vi "Ctor.vi"(8 "error in (no error)":errorcluster) -> (0 "error out":errorcluster, 3 "ByRef Example out":refnum<class "ByRef Example.lvclass">)   [LabVIEW 2012, in "ByRef Example.lvclass"]
uses:
  ByRef Example.lvclass
  Ref Data.ctl
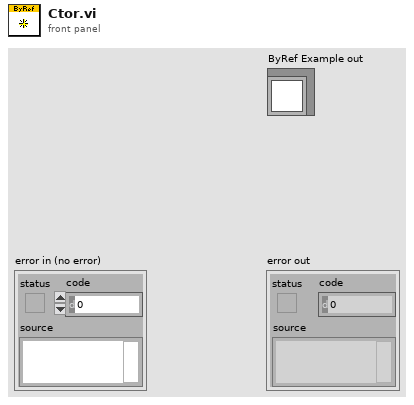
[diagram p1: front panel]
types:
  T1 = typedef "ByRef Example.lvclass/Ref Data.ctl" = cluster{"Boolean":bool, "Numeric":dbl, "String":string}
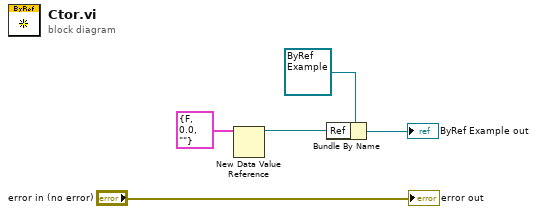
[diagram p0: block diagram]
diagram:
  n1 = New Data Value Reference(data value=T1 {"Boolean"=FALSE, "Numeric"=0.0, "String"=""} ("Ref Data")) -> (data value reference=w1:refnum<data-value>)  [unwired: 1 in, 1 out]
  n2 = Bundle By Name(cluster=refnum<class "ByRef Example.lvclass"> refnum ("ByRef Example in"), "Ref"=w1) -> (→"ByRef Example out":refnum<class "ByRef Example.lvclass">)
  "error out" <- "error in (no error)"
